vi "Open VI FP.vi"(6 "state (Standard)":T1(ring)=enum."Standard", 8 "error in":errorcluster, 9 "open all VI panels? (F)":bool, 10 "VI name":string, 11 "state in":T2) -> (0 "error out":errorcluster, 3 "state out":T2)   [LabVIEW 2010, in "NI_SE_Config Front Panel Layout.lvlib"]
uses:
  NI_SE_Config Front Panel Layout.lvlib
  State.ctl
  VI Info.ctl
  VI Panel Layout/VI Panel Layout.lvclass
  Get VI Info Index by Name.vi
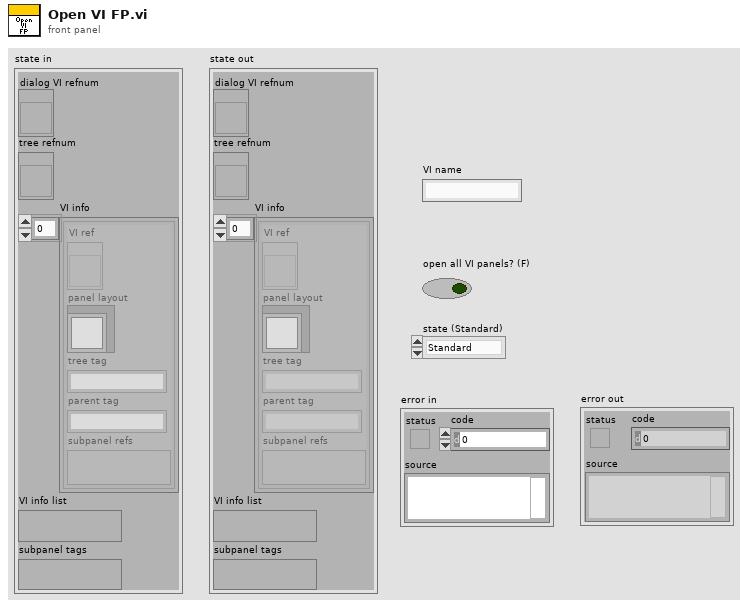
[diagram p1: front panel]
types:
  T1 = enum32{"Invalid", "Standard", "Closed", "Hidden", "Minimized", "Maximized"}
  T2 = typedef "NI_SE_Config Front Panel Layout.lvlib/State.ctl" = cluster{"dialog VI refnum":refnum<vi>, "tree refnum":refnum<vi>, "VI info":T3[], "VI info list":variant, "subpanel tags":variant}
  T3 = typedef "NI_SE_Config Front Panel Layout.lvlib/VI Info.ctl" = cluster{"VI ref":refnum<vi>, "panel layout":refnum<class "VI Panel Layout.lvclass">, "tree tag":string, "parent tag":string, "subpanel refs":variant}
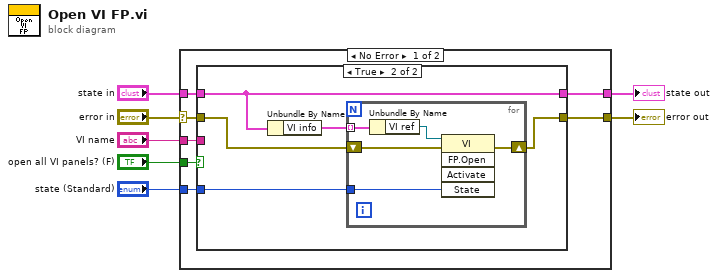
[diagram p0: block diagram]
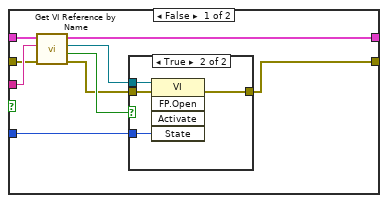
[diagram p2: hidden frame]
diagram:
  n1 = case shown="No Error" "error in" {
    selector: "error in" -> [w13 w39]
    tunnel: "state in" -> [w14 w40]
    tunnel: [w10 w40] -> w5
    tunnel: [w11 w39] -> w4
    tunnel: "VI name" -> [w12 _]
    tunnel: "open all VI panels? (F)" -> [w9 _]
    tunnel: "state (Standard)" -> [w8 _]
    frame No Error {
      n2 = case shown="True" w9 {
        tunnel: w14 -> [w21 w32]
        tunnel: w13 -> [w15 w31]
        tunnel: w12 -> [w20 _]
        tunnel: [w23 w30] -> w11
        tunnel: [w17 w32] -> w10
        tunnel: w8 -> [w22 w29]
        frame False {
          n3 = call "Get VI Reference by Name.vi"("error in"=w15, "VI name"=w20, "state in"=w21) -> ("error out"=w16:errorcluster, "found?"=w18:bool, "VI ref"=w19:refnum<vi>, "state out"=w17:T2)  [unwired: 5 in]
          n4 = case shown="True" w18 {
            tunnel: w16 -> [w24 w28]
            tunnel: [w24 w27] -> w23
            tunnel: w22 -> [_ w26]
            tunnel: w19 -> [_ w25]
            frame False {
            }
            frame True {
              n5 = invoke class="VI" method="FP.Open"(reference=w25, error in=w28, "State"=w26) -> (error out=w27:errorcluster)  [unwired: 2 in, 4 out]
            }
          }
        }
        frame True {
          n6 = Unbundle By Name(w32) -> ("VI info"=w33:T3[])
          n7 = for {
            tunnel: w33 -> [w38] mode=indexing
            shift-right: [w35] -> w30
            shift-left: w31 -> [w36]
            tunnel: w29 -> [w34]
            n8 = Unbundle By Name(w38) -> ("VI ref"=w37:refnum<vi>)
            n9 = invoke class="VI" method="FP.Open"(reference=w37, error in=w36, "State"=w34) -> (error out=w35:errorcluster)  [unwired: 2 in, 4 out]
          }
        }
      }
    }
    frame Error {
    }
  }
  "state out" <- w5
  "error out" <- w4
